vi "BRig_dataCurrent_L_Cue2_T_start_l1.vi"() -> (2 "outputL_Cue2_T_start_l1":i32)   [LabVIEW 2014]
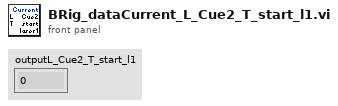
[diagram p1: front panel]
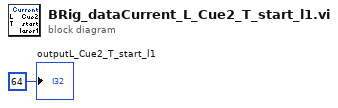
[diagram p0: block diagram]
diagram:
  "outputL_Cue2_T_start_l1" <- 64 ("output_iBlock")
